vi "InitGame.vi"(7 "VI Refnum":refnum<vi>) -> (0 "Error Out":errorcluster={"status"=TRUE, "code"=1026, "source"="Invoke Node in InitGame.vi"}, 3 "MainDataOut":T1={"Image"={"image type"=0, "image depth"=32, "image"=array[640000 elements], "mask"=array[20000 elements], "colors"=[], "Rectangle"={"left"=0, "top"=0, "right"=400, "bottom"=400}}, " TmpImage"={"image type"=0, "image depth"=32, "image"=array[640000 elements], "mask"=array[20000 elements], "colors"=[], "Rectangle"={"left"=0, "top"=0, "right"=400, "bottom"=400}}, "BGColor"=15256322, "FGColor"=13283586, "DRColor"=13283586, "Picture"=bytes[500030], "Queue "=refnum, "EndGameEvent"=refnum, "AnalizeMove"=FALSE})   [LabVIEW 2020]
doc: "Run as pop up with information and basic settings. Initialize game - prepare picture and configuration for next modules."
uses:
  typeDef/MainDataCluster.ctl
  <vilib>/picture/picture.llb/imagedata.ctl
  typeDef/StateMachineEnum.ctl
  typeDef/EventData.ctl
  typeDef/EndType.ctl
  <vilib>/numeric/Random Number (Range) U64.vi
  41e5e3ef-989e-4fef-9c39-9d9951961d26.vi
  <vilib>/numeric/sub_Random U32.vi
  <vilib>/Utility/error.llb/Error Cluster From Error Code.vi
  <vilib>/ErrorRing/Error Ring.xnode
panel:
  in  "Difficulty/Time":dbl(slide)=45.0 scale=30.0..60.0
  in  "Play":bool
  # "Zasady gry"
  # "Celem gry jest odrysowanie \nwylosowanego kształtu."
  # "W zależności od trudności \nwystepuje odpowiedni limit czasowy."
  # "Odrysowanie aktywowane jest \nprzytrzymaniem LPM,\npuszczenie LPM skutkuje zakończeniem\ngry."
  # "Przecięcie/zamknięcie\n narysowanego konturu skutkuje zakończeniem\ngry."
  # "Wyjście poza kontur skutkuje\neliminacją gracza !"
  # "Niedokładne obrysowanie skutkuje\neliminacją gracza !"
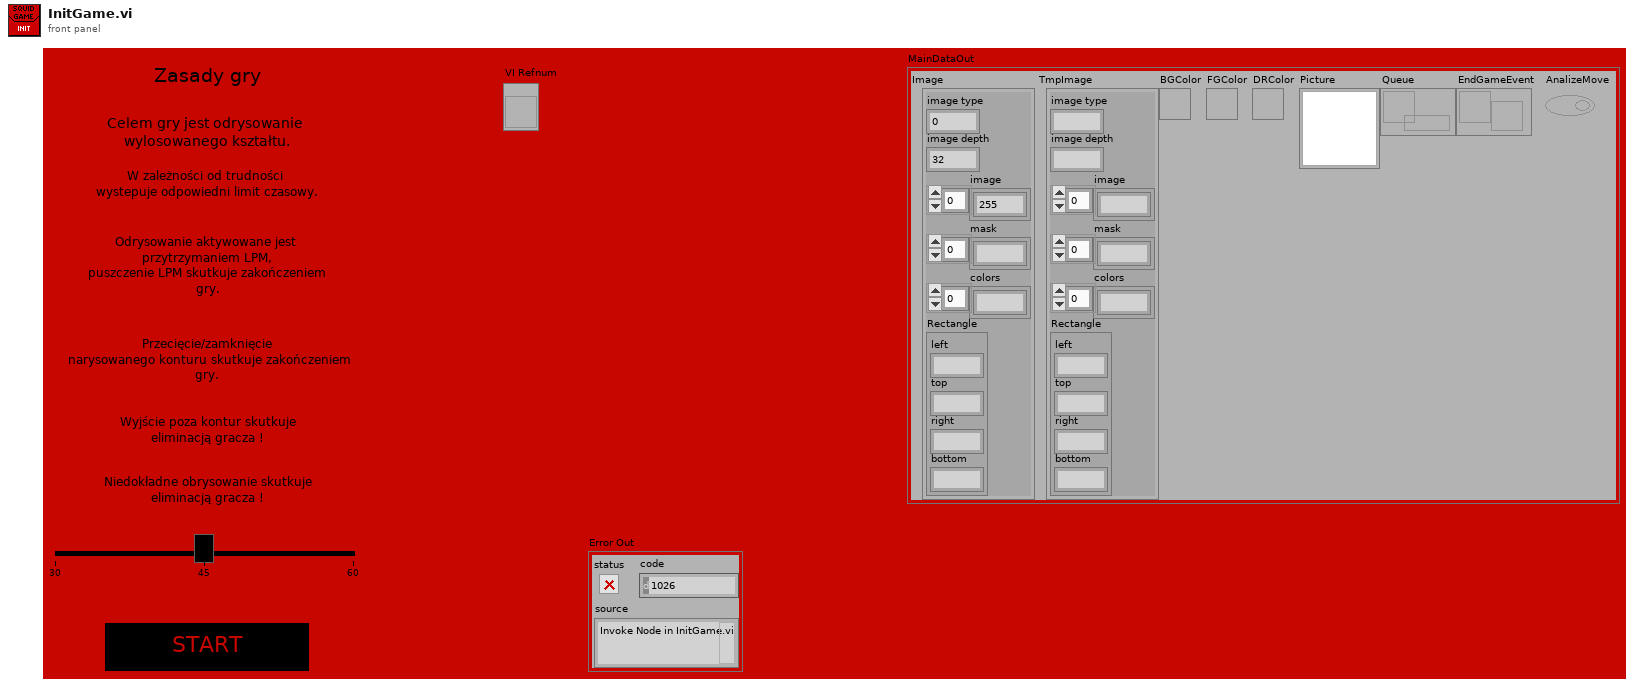
[diagram p1: front panel]
types:
  T1 = typedef "MainDataCluster.ctl" = cluster{"Image":T2, " TmpImage":T2, "BGColor":u32, "FGColor":u32, "DRColor":u32, "Picture":picture, "Queue ":refnum<queue>, "EndGameEvent":refnum<user-event>, "AnalizeMove":bool}
  T2 = typedef "imagedata.ctl" = cluster{"image type":i32, "image depth":i32, "image":u8[], "mask":u8[], "colors":u32[], "Rectangle":cluster{"left":i16, "top":i16, "right":i16, "bottom":i16}}
  T3 = typedef "EventData.ctl" = cluster{"ShowResult":bool, "EndingType":T4}
  T4 = typedef "EndType.ctl" = enum16{"Timeout", "MouseUp", "OutOfLine", "CloseLine", "UserEnd"}
  T5 = typedef "StateMachineEnum.ctl" = enum16{"Init", "ReadTime", "StartTimer", "Result", "StopTimer", "ErrorHandler", "Close"}
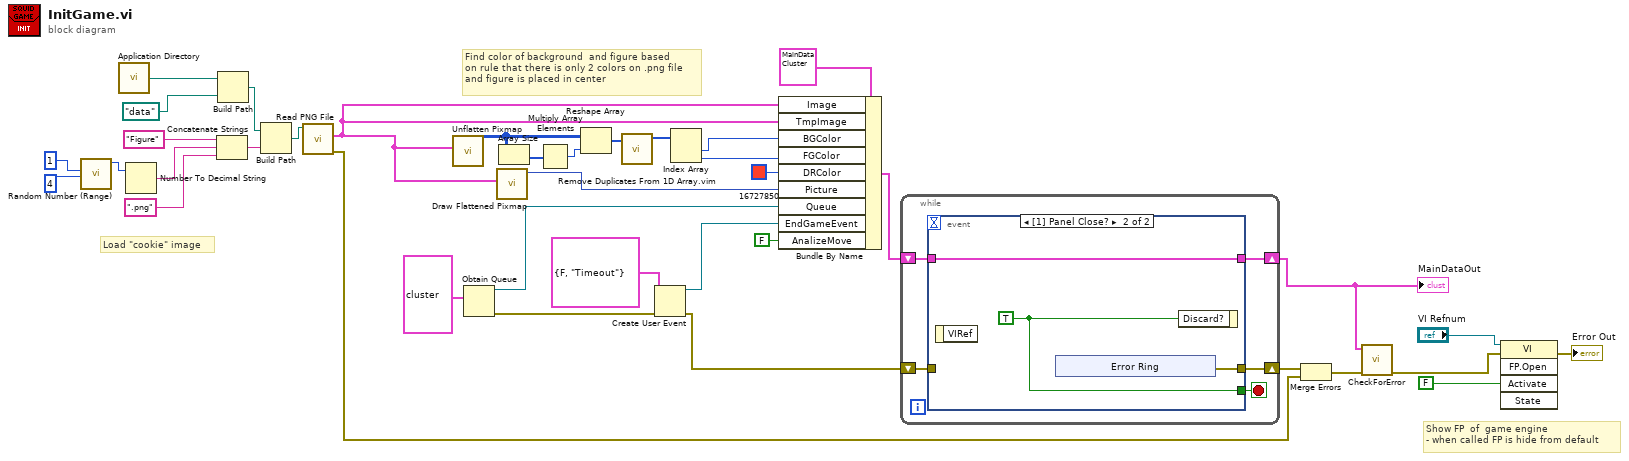
[diagram p0: block diagram]
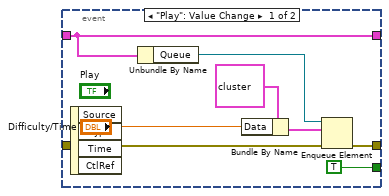
[diagram p2: hidden frame]
diagram:
  # "Load \"cookie\" image"
  # "Show FP  of  game engine\n- when called FP is hide from default"
  # "Find color of background  and figure based\non rule that there is only 2 colors on .png file\nand figure is placed in center"
  n1 = call-poly <vilib>:"Random Number (Range).vi"("lower bound (0)"=u64 1, "upper bound (100)"=u64 4) -> ("number"=w18:u64)  [unwired: 9 in]
  n2 = call <vilib>:"Application Directory.vi"() -> ("Application Directory"=w38:path)
  n3 = Number To Decimal String(number=w18) -> (decimal integer string=w16:string)  [unwired: 1 in]
  n4 = Concatenate Strings("Figure" ("string"), w16, ".png" ("string")) -> (w21:string)
  n5 = Build Path(base path=w38, name or relative path=path "data") -> (appended path=w5:path)
  n6 = Build Path(base path=w5, name or relative path=w21) -> (appended path=w37:path)
  n7 = call <vilib>:"Read PNG File.vi"("path to PNG file"=w37) -> ("error out"=w2:errorcluster, "image data"=w25:T2)  [unwired: 8 in, 1 out]
  n8 = call <vilib>:"Unflatten Pixmap.vi"("image data"=w25) -> ("24-bit pixmap"=w34:u32[][])  [unwired: 4 in, 6 out]
  n9 = Obtain Queue(element data type=cluster{"Data":variant, "State":T5} {"Data"=variant, "State"=enum."Init"}) -> (queue out=w14:refnum<queue>, error out=w13:errorcluster)  [unwired: 4 in, 1 out]
  n10 = call <vilib>:"Draw Flattened Pixmap.vi"("image data"=w25) -> ("new picture"=w28:picture)  [unwired: 8 in]
  n11 = Array Size(array=w34) -> (size(s)=w33:i32[])
  n12 = Multiply Array Elements(1:w33) -> (0:w32:i32)
  n13 = Reshape Array(w34, w32) -> (w31:u32[])
  n14 = call "Remove Duplicates From 1D Array.vim"("array"=w31) -> ("array with duplicates removed"=w30:u32[])  [unwired: 10 in]
  n15 = Create User Event(user event datatype=T3 {"ShowResult"=FALSE, "EndingType"=enum."Timeout"} ("EndData"), error in=w13) -> (user event=w8:refnum<user-event>, error out=w12:errorcluster)
  n16 = Index Array(array=w30) -> (element #1=w26:u32, element #2=w27:u32)  [unwired: 2 in]
  n17 = Bundle By Name(cluster=T1 {"Image"={"image type"=0, "image depth"=32, "image"=array[640000 elements], "mask"=array[20000 elements], "colors"=[], "Rectangle"={"left"=0, "top"=0, "right"=400, "bottom"=400}}, " TmpImage"={"image type"=0, "image depth"=32, "image"=array[640000 elements], "mask"=array[20000 elements], "colors"=[], "Rectangle"={"left"=0, "top"=0, "right"=400, "bottom"=400}}, "BGColor"=15256322, "FGColor"=13283586, "DRColor"=13283586, "Picture"=bytes[500030], "Queue "=refnum, "EndGameEvent"=refnum, "AnalizeMove"=FALSE}, "Image"=w25, "TmpImage"=w25, "BGColor"=w26, "FGColor"=w27, "DRColor"=u32 16727850, "Picture"=w28, "Queue"=w14, "EndGameEvent"=w8, "AnalizeMove"=FALSE) -> (w11:T1)
  n18 = while {
    shift-right: [w42] -> w10
    shift-left: w12 -> [w43]
    shift-right: [w39] -> w6
    shift-left: w11 -> [w40]
    stop <- w41 stop-if-true
    n19 = event shown="[1] Panel Close?" {
      selector: _ -> [_ _]
      dyn-events: _ -> [_ _]
      timeout: _ -> [_ _]
      tunnel: w43 -> [w51 _]
      tunnel: [w49 w52] -> w42
      tunnel: [TRUE w54] -> w41
      tunnel: w40 -> [w47 w53]
      tunnel: [w47 w53] -> w39
      event "Play": Value Change {
        n20 = event-data() -> ()  [unwired: 1 in, 4 out]
        n21 = Unbundle By Name(w47) -> ("Queue"=w48:refnum<queue>)
        n22 = Bundle By Name(cluster=cluster{"Data":variant, "State":T5} {"Data"=variant, "State"=enum."Init"} ("element"), "Data"="Difficulty/Time") -> (w45:cluster{"Data":variant, "State":T5})
        n23 = Enqueue Element(queue=w48, element=w45, error in (no error)=w51) -> (error out=w49:errorcluster)  [unwired: 1 in, 2 out]
      }
      event Panel Close? {
        w54 = TRUE
        n24 = event-data() -> ()  [unwired: 1 in, 1 out]
        n25 = xnode "Error Ring"() -> ("error out"=w52:errorcluster)
        n26 = event-data("Discard?"=w54) -> ()  [unwired: 1 in, 1 out]
      }
    }
  }
  "MainDataOut" <- w6
  n27 = Merge Errors(w10, w2) -> (w3:errorcluster)
  n28 = call "CheckForError.vi"("Error In"=w3, "MainData In"=w6) -> ("Error Out"=w7:errorcluster)  [unwired: 9 in]
  n29 = invoke class="VI" method="FP.Open"(reference="VI Refnum", error in=w7, "Activate"=FALSE ("Activate?")) -> (error out=→"Error Out":errorcluster)  [unwired: 2 in, 4 out]
